vi "Process.vi"(8 "error in (no error)":errorcluster, 11 "Process In":refnum<class "Debug View.lvclass">) -> (0 "error out":errorcluster, 3 "Process Out":refnum<class "Debug View.lvclass">)   [LabVIEW 2020]
uses:
  Debug View.lvclass
  Debug View.lvclass/Debug View.ctl
  <vilib>/Utility/error.llb/Clear Errors.vi
  <vilib>/Utility/error.llb/Error Cluster From Error Code.vi
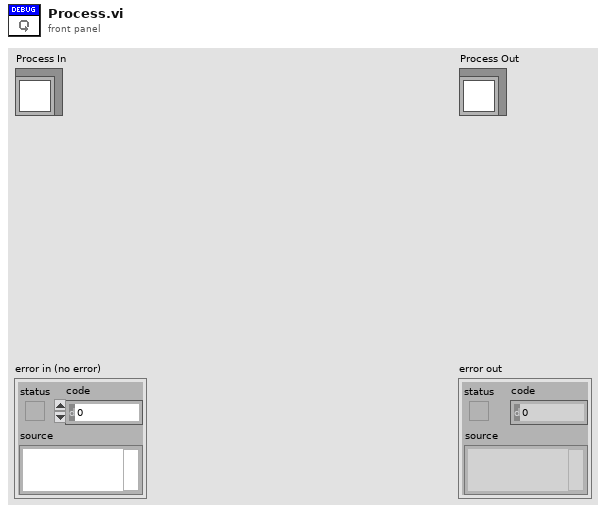
[diagram p1: front panel]
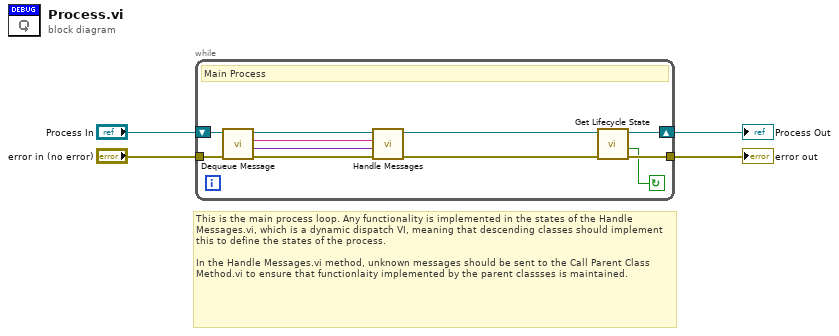
[diagram p0: block diagram]
diagram:
  # "This is the main process loop. Any functionality is implemented in the states of the Handle Messages.vi, which is a dynamic dispatch VI, meaning that descending classes should implement this to define the states of the process.\n\nIn the Handle Messages.vi method, unknown messages should be sent to the Call Parent Class Method.vi to ensure that functionlaity implemented by the parent classses is maintained."
  n1 = while {
    shift-right: [w6] -> w3
    shift-left: "Process In" -> [w15]
    tunnel: "error in (no error)" -> [w14]
    tunnel: [w7] -> w1
    stop <- w5 continue-if-true
    # "Main Process"
    n2 = call "Dequeue Message.vi"("error in (no error)"=w14, "Process In"=w15) -> ("error out"=w11:errorcluster, "Message Data"=w9:variant, "Message"=w10:string, "Process Out"=w12:refnum<class "Debug View.lvclass">)  [unwired: 6 in]
    n3 = call-dynamic "Handle Messages.vi"("error in (no error)"=w11, "Message Data"=w9, "Message"=w10, "Process In"=w12) -> ("error out"=w13:errorcluster, "Process Out"=w8:refnum<class "Debug View.lvclass">)  [unwired: 6 in]
    n4 = call "Get Lifecycle State.vi"("error in (no error)"=w13, "Process In"=w8) -> ("error out"=w7:errorcluster, "In Process Loop?"=w5:bool, "Process Out"=w6:refnum<class "Debug View.lvclass">)  [unwired: 6 in, 1 out]
  }
  "error out" <- w1
  "Process Out" <- w3
